vi "Debug_Convert_Data_to_String.vi"(8 "error in (no error)":errorcluster, 11 "AB_Source_ExportedVI in":refnum<class "AB_Source_ExportedVI.lvclass">) -> (0 "error out":errorcluster, 1 "classData":string, 2 "sourceType":string, 3 "AB_Source_ExportedVI out":refnum<class "AB_Source_ExportedVI.lvclass">)   [LabVIEW 2020, in "AB_Source_ExportedVI.lvclass"]
uses:
  <vilib>/AppBuilder/AB_Classes/Source/ExportedVI/AB_Source_ExportedVI.lvclass
  <vilib>/AppBuilder/AB_Classes/Source/ExportedVI/AB_Source_ExportedVI.lvclass/AB_Source_ExportedVI.ctl
  <vilib>/AppBuilder/AB_Classes/Source/VI/AB_Source_VI.lvclass
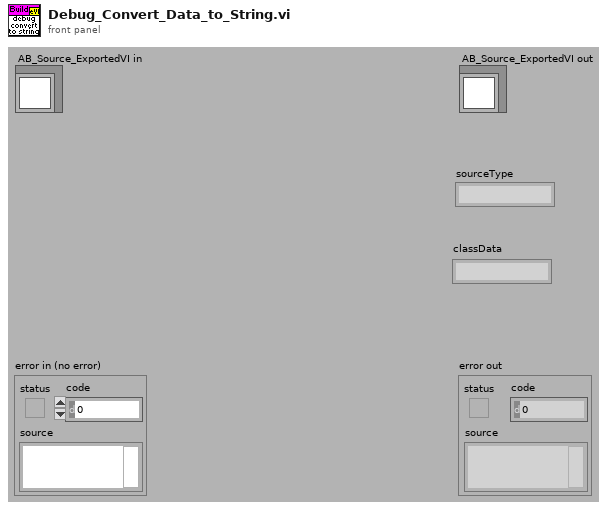
[diagram p1: front panel]
types:
  T1 = cluster{"name":string, "dir":enum32{"in", "out", "in/out", "length", "error-out"}, "inputIdx":i32, "outputIdx":i32, "passBy":i32, "lenInput":i32, "lenOutput":i32}[]
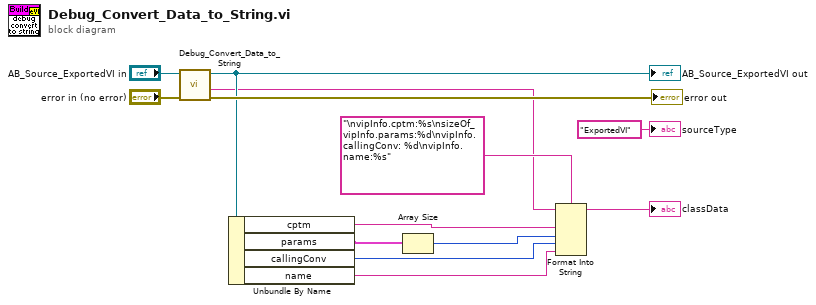
[diagram p0: block diagram]
diagram:
  n1 = call-parent "Debug_Convert_Data_to_String.vi"("error in (no error)"="error in (no error)", "AB_Source_VI in"="AB_Source_ExportedVI in") -> ("error out"=→"error out":errorcluster, "classData"=w7:string, "AB_Source_VI out"=w9:refnum<class "AB_Source_ExportedVI.lvclass">)  [unwired: 6 in, 1 out]
  "AB_Source_ExportedVI out" <- w9
  n2 = Unbundle By Name(w9) -> ("cptm"=w5:string, "params"=w4:T1, "callingConv"=w2:i32, "name"=w1:string)
  n3 = Array Size(array=w4) -> (size(s)=w3:i32)
  n4 = Format Into String(format string="\nvipInfo.cptm:%s\nsizeOf_vipInfo.params:%d\nvipInfo.callingConv: %d\nvipInfo.name:%s", initial string=w7, w5, w3, w2, w1) -> (resulting string=→"classData":string)  [unwired: 1 in, 1 out]
  "sourceType" <- "ExportedVI" ("sourceType")
